vi "插件.vi"() -> ()   [LabVIEW 2011]
panel:
  in  "stop":bool
  in  "X":dbl
  in  "Y":dbl
  out "output":dbl
  in  "Ring 2":u16(ring) items=["Add.vi", "Divide.vi", "Max.vi", "Mean.vi", "Multiple.vi", "Subtract.vi", "Untitled 2.vi"]
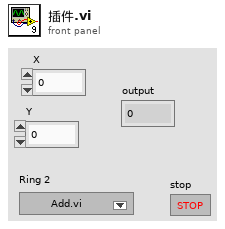
[diagram p1: front panel]
types:
  T1 = enum32{"invalid app kind", "Development System", "Run Time System", "Student Edition", "Embedded LabVIEW", "Evaluation", "Custom"}
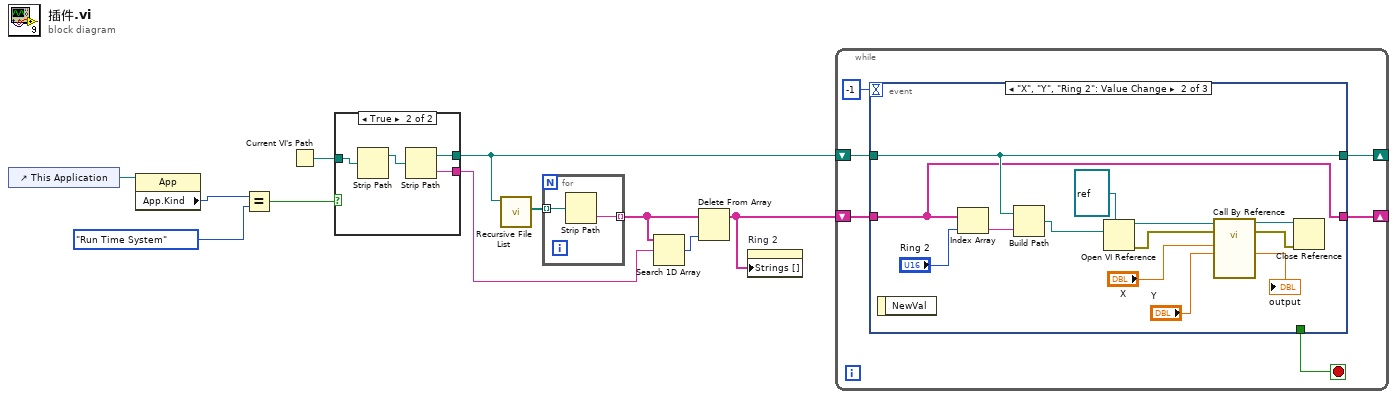
[diagram p0: block diagram]
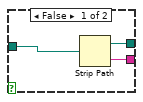
[diagram p2: hidden frame]
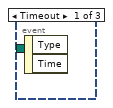
[diagram p3: hidden frame]
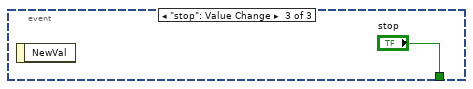
[diagram p4: hidden frame]
diagram:
  n1 = control-ref of="This Application"() -> (w4:refnum<vi>)
  n2 = property class="App"(reference=w4) -> ("App.Kind"=w3:T1)  [unwired: 1 in, 2 out]
  n3 = Equal?(x=w3, y=T1."Run Time System" ("Application:Kind")) -> (x = y?=w1:bool)
  n4 = Current VI's Path() -> (path=w11:path)
  n5 = case shown="True" w1 {
    tunnel: w11 -> [w14 w16]
    tunnel: [w13 w18] -> w10
    tunnel: [w12 w17] -> w6
    frame False {
      n6 = Strip Path(path=w14) -> (stripped path=w13:path, name=w12:string)
    }
    frame True {
      n7 = Strip Path(path=w16) -> (stripped path=w15:path)  [unwired: 1 out]
      n8 = Strip Path(path=w15) -> (stripped path=w18:path, name=w17:string)
    }
  }
  n9 = call <vilib>:"Recursive File List.vi"("Folder Path"=w10) -> ("All Files in Dir"=w9:path[])  [unwired: 6 in, 4 out]
  n10 = for {
    tunnel: [w20] -> _ mode=indexing
    tunnel: w9 -> [w20] mode=indexing
    tunnel: [w19] -> w7 mode=indexing
    n11 = Strip Path(path=w20) -> (name=w19:string)  [unwired: 1 out]
  }
  n12 = Search 1D Array(1D array=w7, element=w6) -> (index of element=w8:i32)  [unwired: 1 in]
  n13 = Delete From Array(array=w7, index=w8) -> (array with subset deleted=w5:string[])  [unwired: 1 in, 1 out]
  n14 = property on="Ring 2" class="Ring (strict)"("Strings []"=w5) -> ()  [unwired: 2 in, 2 out]
  n15 = while {
    shift-right: [w25] -> _
    shift-left: w10 -> [w26]
    shift-right: [w21] -> _
    shift-left: w5 -> [w22]
    stop <- w24 stop-if-true
    n16 = event shown="[1] \"X\", \"Y\", \"Ring 2\": Value Change" {
      selector: _ -> [_ _ _]
      dyn-events: _ -> [_ _ _]
      timeout: -1 -> [_ _ _]
      tunnel: w26 -> [_ w39 _]
      tunnel: [_ w39 _] -> w25
      tunnel: [_ _ "stop"] -> w24
      tunnel: w22 -> [_ w28 _]
      tunnel: [_ w28 _] -> w21
      event Timeout {
        n17 = event-data() -> ()  [unwired: 1 in, 2 out]
      }
      event "X", "Y", "Ring 2": Value Change {
        n18 = event-data() -> ()  [unwired: 1 in, 1 out]
        n19 = Index Array(array=w28, index="Ring 2") -> (element=w27:string)
        n20 = Build Path(base path=w39, name or relative path=w27) -> (appended path=w38:path)
        n21 = Open VI Reference(type specifier VI Refnum (for type only)=refnum<vi> refnum, vi path=w38) -> (vi reference=w37:refnum<vi>, error out=w36:errorcluster)  [unwired: 4 in]
        n22 = call-by-ref "?"(reference=w37, error in=w36, "input2"="Y", "input1"="X") -> (reference out=w35:refnum<vi>, error out=w34:errorcluster, "output"=→"output":dbl)  [unwired: 8 in, 1 out]
        n23 = Close Reference(reference=w35, error in (no error)=w34) -> ()  [unwired: 1 out]
      }
      event "stop": Value Change {
        n24 = event-data() -> ()  [unwired: 1 in, 1 out]
      }
    }
  }
